vi "MultipleLinesToPoints.vi"(4 "Sim":bool, 5 "mode":enum16{"Manual", "Quad", "Vertical", "Half"}(ring), 6 "Arc Threshold":dbl, 7 "Least Dis":dbl, 8 "holder_length":dbl, 9 "lines":string[](array[string])) -> (0 "InRange":bool, 1 "y":dbl[](array[numeric]), 2 "z":dbl[](array[numeric]), 3 "x":dbl[](array[numeric]))   [LabVIEW 2013]
uses:
  <vilib>/Native 3D Graph/xcontrol/3DPC_SurfacePlot.xctl
  <vilib>/Analysis/_algsub.llb/Real Vector Norm.vi
  <vilib>/Analysis/NI_AALPro.lvlib
  <vilib>/Platform/NI_3dgraph.lvlib
panel:
  out "output cluster":cluster{dbl, i32, dbl, i32}
  in  "theta2_open":dbl
  in  "3D Curve - Lorenz Attractor":refnum<k7>(container)
  out "size(s)":i32
  out "x+y":dbl[](array[numeric])
  in  "milliseconds to wait":u32
  out "Test Graph Graph Real Time":refnum<class "Base Datatype.lvclass">[](xcontrol)
  out "x":dbl[](array[numeric])
  out "theta2":dbl[](array[numeric])
  out "theta1":dbl[](array[numeric])
  in  "file path (use dialog)":path=path "E:/Dropbox/StaredProject/Distributed3D/D3DM/sim_input.txt"
  out "filteredLine":string[](array[string])
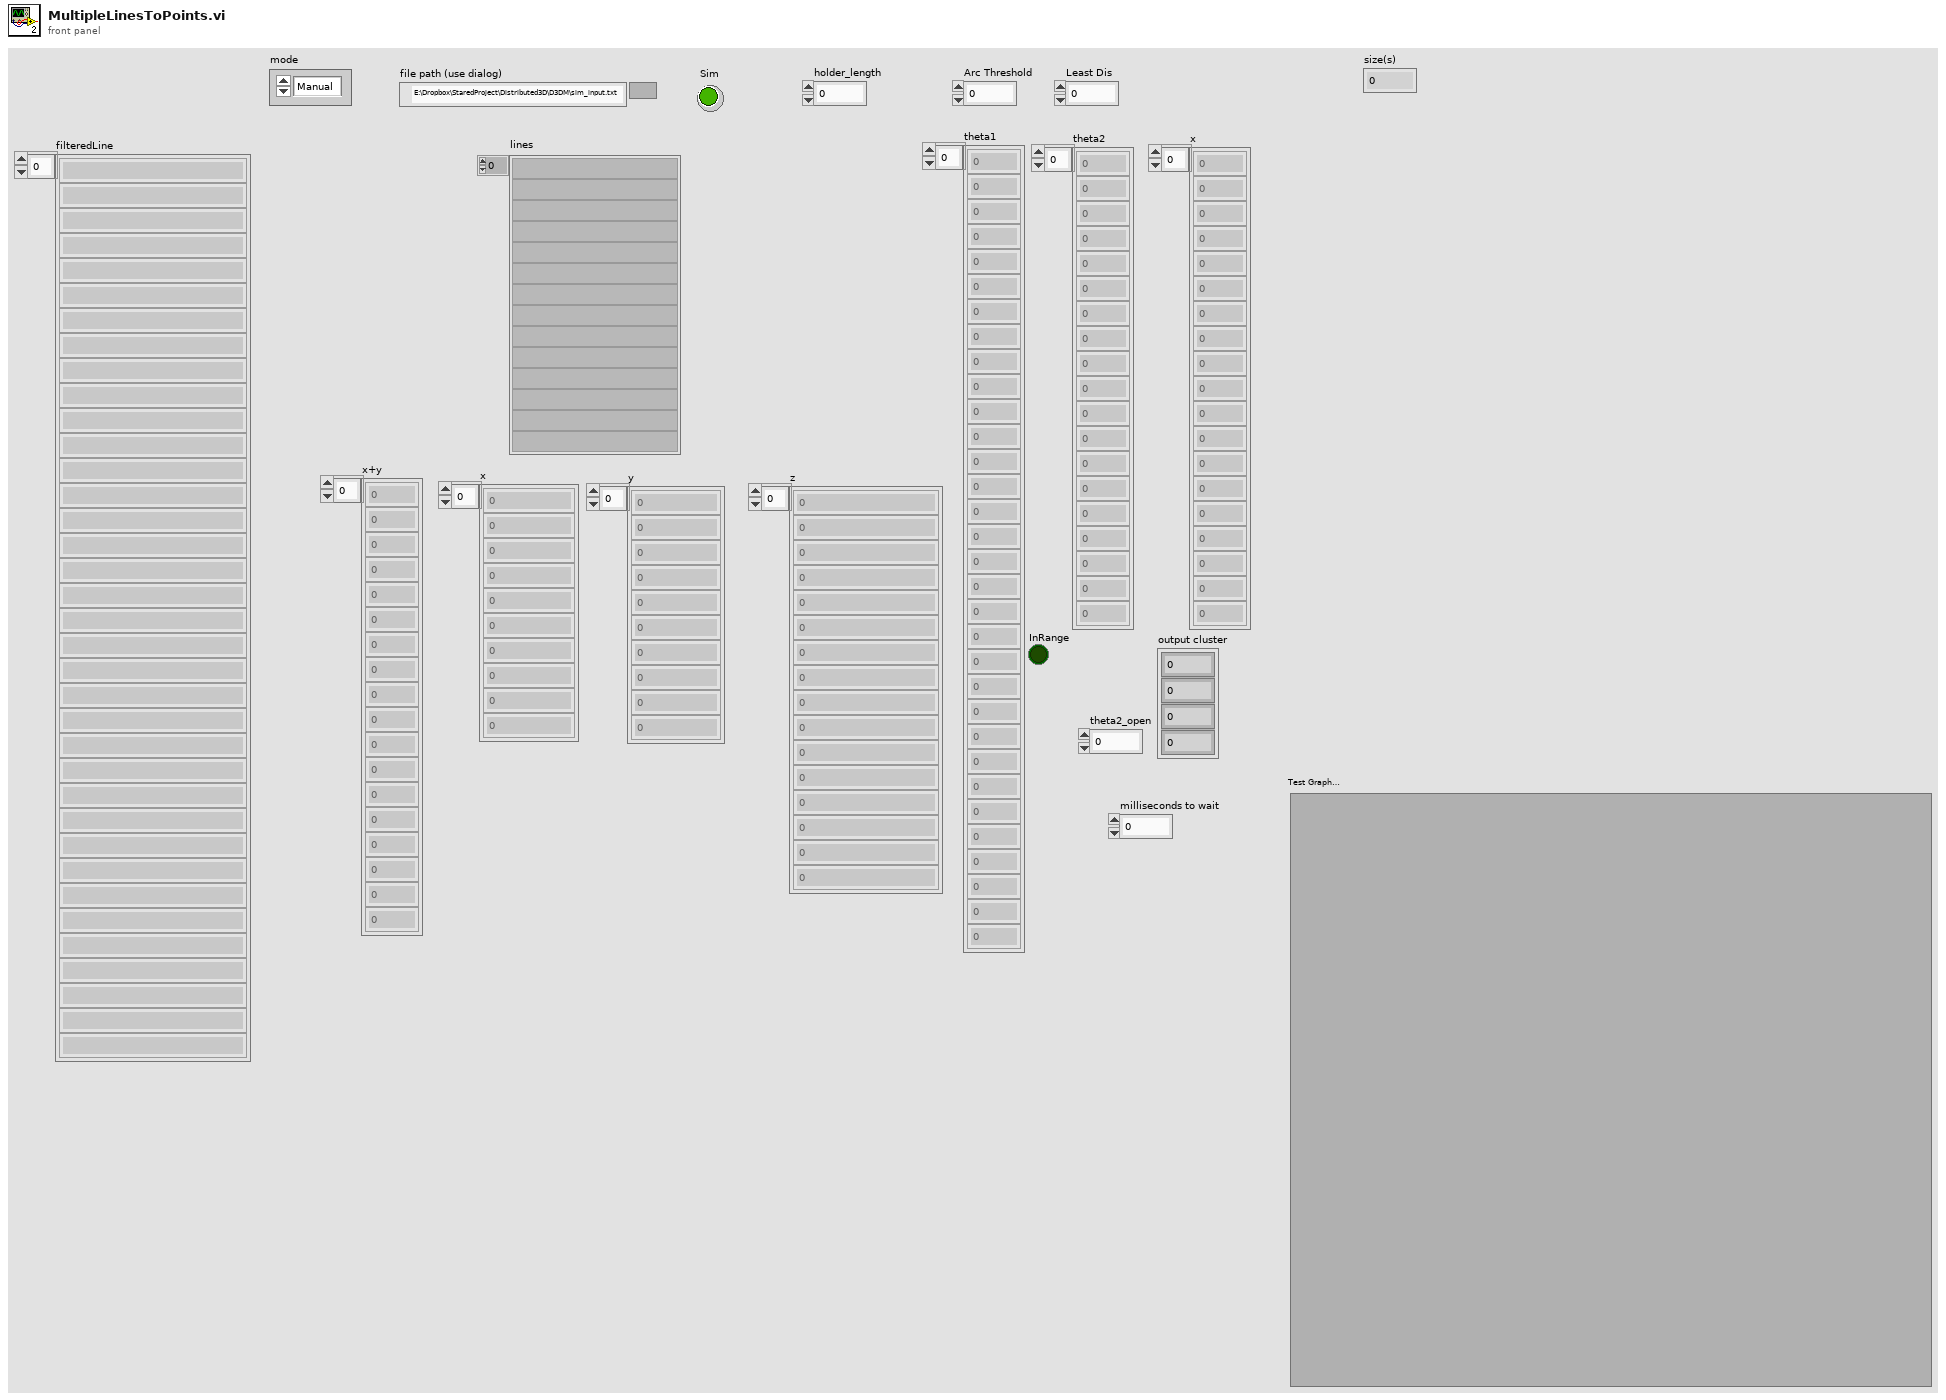
[diagram p1: front panel]
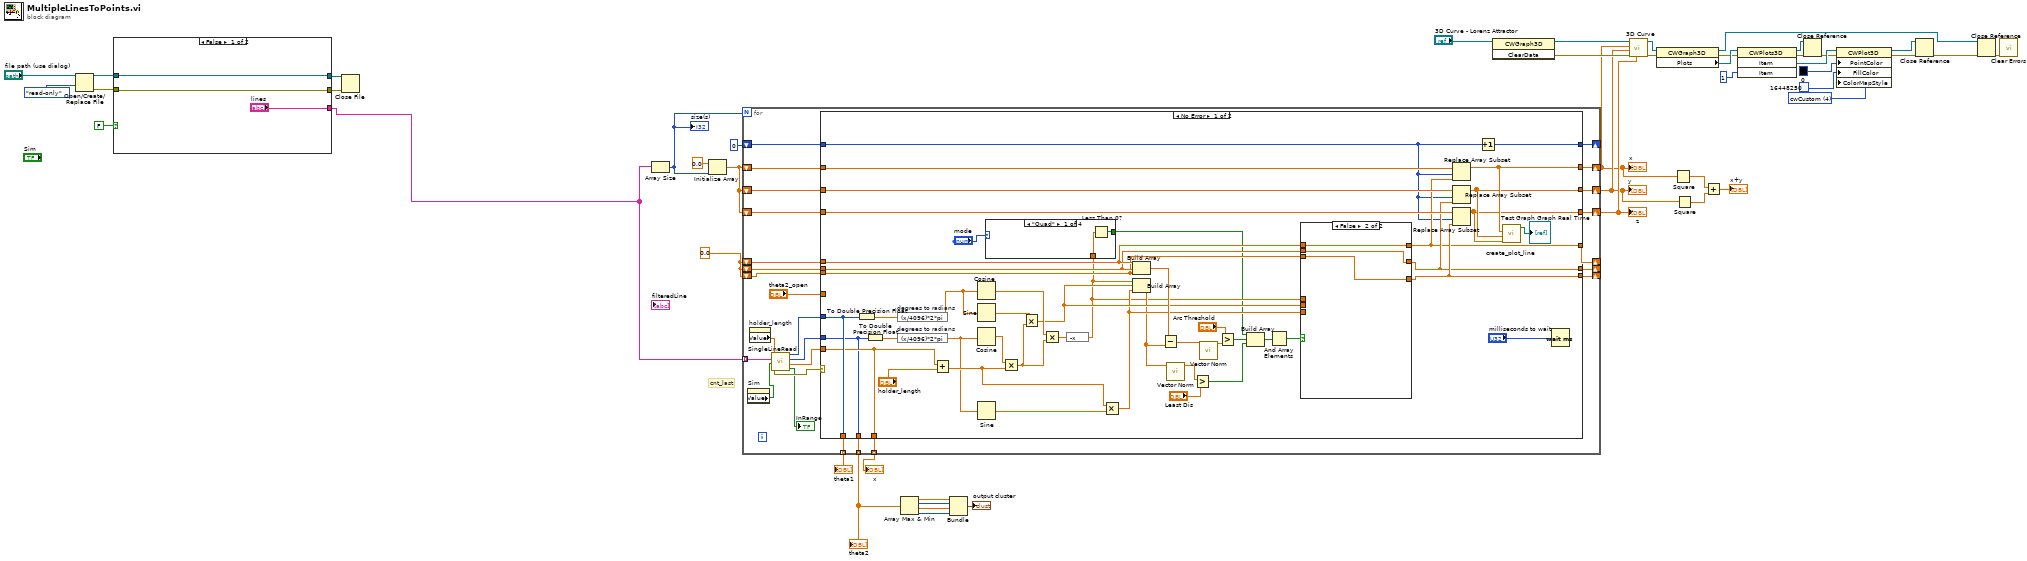
[diagram p0: block diagram]
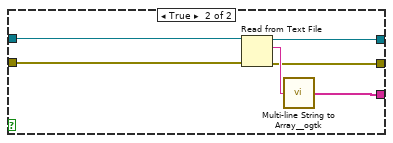
[diagram p2: hidden frame]
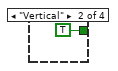
[diagram p3: hidden frame]
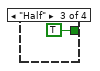
[diagram p4: hidden frame]
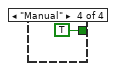
[diagram p5: hidden frame]
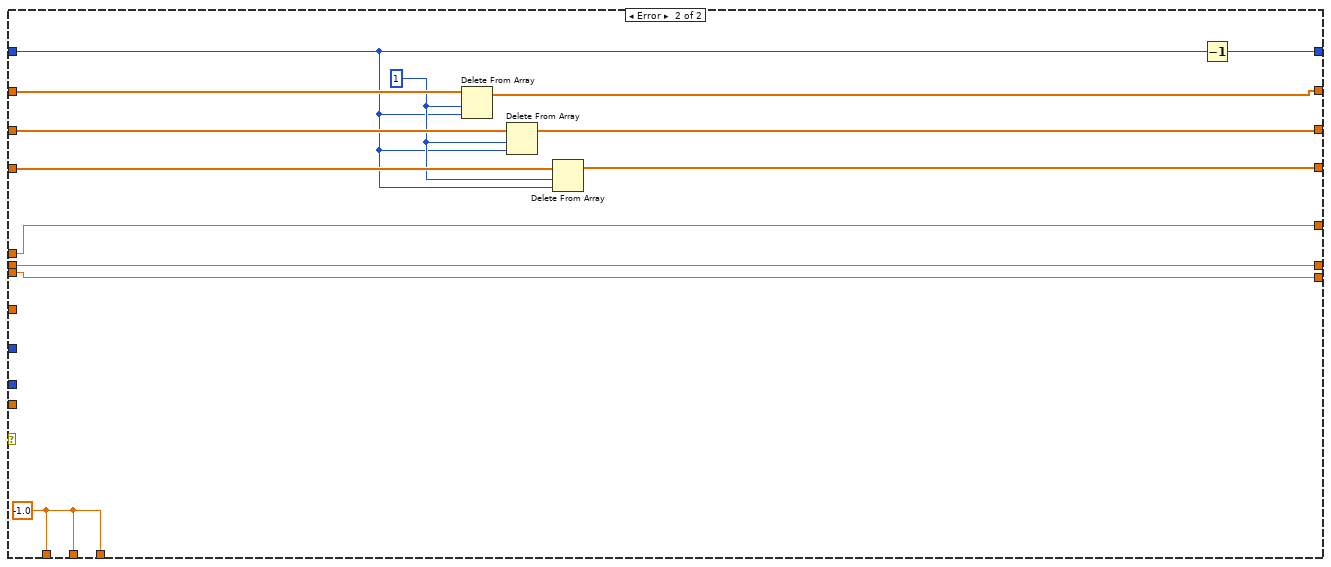
[diagram p7: hidden frame]
diagram:
  w17 = 4 items=["cwNone", "cwShaded", "cwColorSpectrum", "cwGrayScale", "cwCustom"] ("ColorMapStyle")
  w35 = 0.0
  # "cnt_last"
  n1 = Open/Create/Replace File(file path (use dialog)="file path (use dialog)", access (0:read/write)=enum16{"read/write", "read-only", "write-only"}."read-only") -> (refnum out=w41:refnum<file>, error out=w40:errorcluster)  [unwired: 4 in, 1 out]
  n2 = case shown="False" FALSE {
    tunnel: ["lines" w55] -> w9
    tunnel: [w49 w54] -> w45
    tunnel: [w48 w53] -> w44
    tunnel: w41 -> [w49 w52]
    tunnel: w40 -> [w48 w51]
    frame False {
    }
    frame True {
      n3 = Read from Text File(file (use dialog)=w52, error in=w51) -> (refnum out=w54:refnum<file>, text=w56:string, error out=w53:errorcluster)  [unwired: 2 in, 1 out]
      n4 = call <userlib>:"Multi-line String to Array__ogtk.vi"("string"=w56) -> ("lines"=w55:string[])
    }
  }
  n5 = Close File(refnum=w45, error in=w44) -> ()  [unwired: 2 out]
  n6 = Array Size(array=w9) -> (size(s)=w10:i32)
  "size(s)" <- w10
  n7 = Initialize Array(0.0 ("element"), w10) -> (w46:dbl[])
  n8 = for {
    N: w10 -> [_]
    shift-right: [w79] -> w12
    shift-left: w46 -> [w82]
    shift-right: [w78] -> w13
    shift-left: w46 -> [w81]
    shift-right: [w77] -> w14
    shift-left: w46 -> [w80]
    tunnel: [w65] -> w39 mode=indexing
    shift-right: [w71] -> _
    shift-left: w35 -> [w76]
    shift-right: [w72] -> _
    shift-left: w35 -> [w75]
    shift-right: [w73] -> _
    shift-left: w35 -> [w74]
    tunnel: w9 -> [w69] mode=indexing
    shift-right: [w66] -> _
    shift-left: 0 -> [w67]
    tunnel: [w64] -> w6 mode=indexing
    tunnel: [w63] -> w7 mode=indexing
    n9 = property on="Sim" class="Bool (strict)"() -> ("Value"=w70:bool)  [unwired: 2 in, 2 out]
    n10 = property on="holder_length" class="DigNum (strict)"() -> ("Value"=w57:dbl)  [unwired: 2 in, 2 out]
    n11 = call "SingleLineRead.vi"("Sim"=w70, "line"=w69, "Holder Length"=w57) -> ("InRange"=→"InRange":bool, "length"=w60:dbl, "armAngle"=w59:i32, "baseAngle"=w58:i32, "error out"=w68:errorcluster)  [unwired: 1 in]
    n12 = case shown="No Error" w68 {
      tunnel: w82 -> [w129 w150]
      tunnel: w81 -> [w128 w149]
      tunnel: w80 -> [w127 w148]
      tunnel: [w125 w146] -> w79
      tunnel: [w124 w145] -> w78
      tunnel: [w123 w144] -> w77
      tunnel: w59 -> [w94 _]
      tunnel: w58 -> [w96 _]
      tunnel: w76 -> [w111 w153]
      tunnel: w75 -> [w110 w152]
      tunnel: w74 -> [w109 w151]
      tunnel: [w105 w151] -> w73
      tunnel: [w104 w152] -> w72
      tunnel: [w103 w153] -> w71
      tunnel: w60 -> [w95 _]
      tunnel: w67 -> [w98 w142]
      tunnel: [w97 w143] -> w66
      tunnel: [w96 w141] -> w65
      tunnel: [w94 w141] -> w64
      tunnel: [w95 w141] -> w63
      tunnel: "theta2_open" -> [_ _]
      frame No Error {
        n13 = To Double Precision Float(number=w96) -> (double precision float=w91:dbl)
        n14 = To Double Precision Float(number=w94) -> (double precision float=w90:dbl)
        n15 = expression code="(x/4096)*2*pi" "degrees to radians"(w91) -> (w121:dbl)
        n16 = expression code="(x/4096)*2*pi" "degrees to radians"(w90) -> (w92:dbl)
        n17 = Add(x=w95, y="holder_length") -> (x+y=w93:dbl)
        n18 = Cosine(x=w121) -> (cos(x)=w117:dbl)
        n19 = Sine(x=w121) -> (sin(x)=w118:dbl)
        n20 = Cosine(x=w92) -> (cos(x)=w119:dbl)
        n21 = Sine(x=w92) -> (sin(x)=w115:dbl)
        n22 = Multiply(x=w119, y=w93) -> (x*y=w116:dbl)
        n23 = Multiply(x=w118, y=w116) -> (x*y=w107:dbl)
        n24 = Multiply(x=w117, y=w116) -> (x*y=w108:dbl)
        n25 = expression code="-x"(w108) -> (w88:dbl)
        n26 = case shown="\"Quad\"" "mode" {
          tunnel: w88 -> [w131 _ _ _]
          tunnel: [w130 TRUE TRUE TRUE] -> w85
          frame "Quad" {
            n27 = Less Than 0?(x=w131) -> (x < 0?=w130:bool)
          }
          frame "Vertical" {
          }
          frame "Half" {
          }
          frame "Manual" {
          }
        }
        n28 = Multiply(x=w93, y=w115) -> (x*y=w106:dbl)
        n29 = Build Array(w111, w110, w109) -> (w112:dbl[])
        n30 = Build Array(w88, w107, w106) -> (w101:dbl[])
        n31 = Subtract(x=w112, y=w101) -> (x-y=w102:dbl[])
        n32 = call-poly <vilib>:"Vector Norm.vi"("Input Vector"=w101) -> ("norm"=w99:dbl)  [unwired: 9 in, 1 out]
        n33 = Greater?(x=w99, y="Least Dis") -> (0:w86:bool)
        n34 = call-poly <vilib>:"Vector Norm.vi"("Input Vector"=w102) -> ("norm"=w114:dbl)  [unwired: 9 in, 1 out]
        n35 = Greater?(x="Arc Threshold", y=w114) -> (0:w87:bool)
        n36 = Build Array(w85, w87, w86) -> (w84:bool[])
        n37 = And Array Elements(Boolean array=w84) -> (logical AND=w83:bool)
        n38 = case shown="False" w83 {
          tunnel: [w137 w140] -> w103
          tunnel: [w136 w139] -> w104
          tunnel: [w135 w138] -> w105
          tunnel: w111 -> [_ w140]
          tunnel: w110 -> [_ w139]
          tunnel: w109 -> [_ w138]
          tunnel: w88 -> [w137 _]
          tunnel: w107 -> [w136 _]
          tunnel: w106 -> [w135 _]
          frame True {
          }
          frame False {
          }
        }
        n39 = Replace Array Subset(array=w129, new element=w103, index=w98) -> (w125:dbl[])
        n40 = Replace Array Subset(array=w128, new element=w104, index=w98) -> (w124:dbl[])
        n41 = Replace Array Subset(array=w127, new element=w105, index=w98) -> (w123:dbl[])
        n42 = Increment(x=w98) -> (x+1=w97:i32)
        n43 = call <vilib>:"create_plot_line.vi"("z vector"=w123, "y vector"=w124, "x vector"=w125) -> ("plots out"=→"Test Graph Graph Real Time":refnum<class "Base Datatype.lvclass">[])  [unwired: 8 in]
        n44 = Wait (ms)(milliseconds to wait="milliseconds to wait") -> ()  [unwired: 1 out]
      }
      frame Error {
        w141 = -1.0
        w147 = 1
        n45 = Delete From Array(array=w150, length=w147, index=w142) -> (array with subset deleted=w146:dbl[])  [unwired: 1 out]
        n46 = Delete From Array(array=w149, length=w147, index=w142) -> (array with subset deleted=w145:dbl[])  [unwired: 1 out]
        n47 = Delete From Array(array=w148, length=w147, index=w142) -> (array with subset deleted=w144:dbl[])  [unwired: 1 out]
        n48 = Decrement(x=w142) -> (x-1=w143:i32)
      }
    }
  }
  "x" <- w12
  "y" <- w13
  "z" <- w14
  "theta1" <- w39
  "theta2" <- w6
  "x" <- w7
  n49 = Array Max & Min(array=w6) -> (max value=w5:dbl, max index (indices)=w4:i32, min value=w3:dbl, min index (indices)=w2:i32)
  n50 = Bundle(w5, w4, w3, w2) -> (→"output cluster":cluster{dbl, i32, dbl, i32})  [unwired: 1 in]
  n51 = invoke class="CWGraph3D" method="ClearData"(reference="3D Curve - Lorenz Attractor") -> (reference out=w16:refnum<k7>, error out=w15:errorcluster)  [unwired: 2 in, 1 out]
  n52 = call <vilib>:"3D Curve.vi"("z vector"=w14, "error in (no error)"=w15, "y vector"=w13, "x vector"=w12, "3D graph"=w16) -> ("error out"=w31:errorcluster, "3D graph out"=w30:refnum<k7>)  [unwired: 5 in]
  n53 = property class="CWGraph3D"(reference=w30, error in=w31) -> (reference out=w21:refnum<k7>, error out=w29:errorcluster, "Plots"=w33:refnum<k7>)
  n54 = Square(x=w12) -> (x^2=w38:dbl[])
  n55 = Square(x=w13) -> (x^2=w37:dbl[])
  n56 = Add(x=w38, y=w37) -> (x+y=→"x+y":dbl[])
  n57 = invoke class="CWPlots3D" method="Item"(reference=w33, error in=w29, "Item"=1) -> (reference out=w27:refnum<k7>, error out=w28:errorcluster, "Item"=w32:refnum<k7>)  [unwired: 1 in, 1 out]
  n58 = Close Reference(reference=w27, error in (no error)=w28) -> (error out=w26:errorcluster)
  n59 = property class="CWPlot3D"(reference=w32, error in=w26, "PointColor"=u32 0, "FillColor"=u32 16448250, "ColorMapStyle"=w17) -> (reference out=w24:refnum<k7>, error out=w25:errorcluster)
  n60 = Close Reference(reference=w24, error in (no error)=w25) -> (error out=w22:errorcluster)
  n61 = Close Reference(reference=w21, error in (no error)=w22) -> (error out=w23:errorcluster)
  n62 = call <vilib>:"Clear Errors.vi"("error in (no error)"=w23) -> ()  [unwired: 6 in, 1 out]
